vi "bgd squarewave.vi"(9 "YScale.Maximum":dbl, 10 "ZScale.Maximum":dbl, 11 "Cond. Intens. 2":dbl[][](graph)) -> (3 "square wave":dbl[][](array[numeric]))   [LabVIEW 2016]
uses:
  <vilib>/Analysis/NI_AALBase.lvlib
panel:
  in  "place on color scale":dbl(slide)=3.25 scale=0.0..10.0
  in  "color difference":dbl(slide)=8.0 scale=0.0..10.0
  out "Cond. Intens. 3":dbl[][](graph)
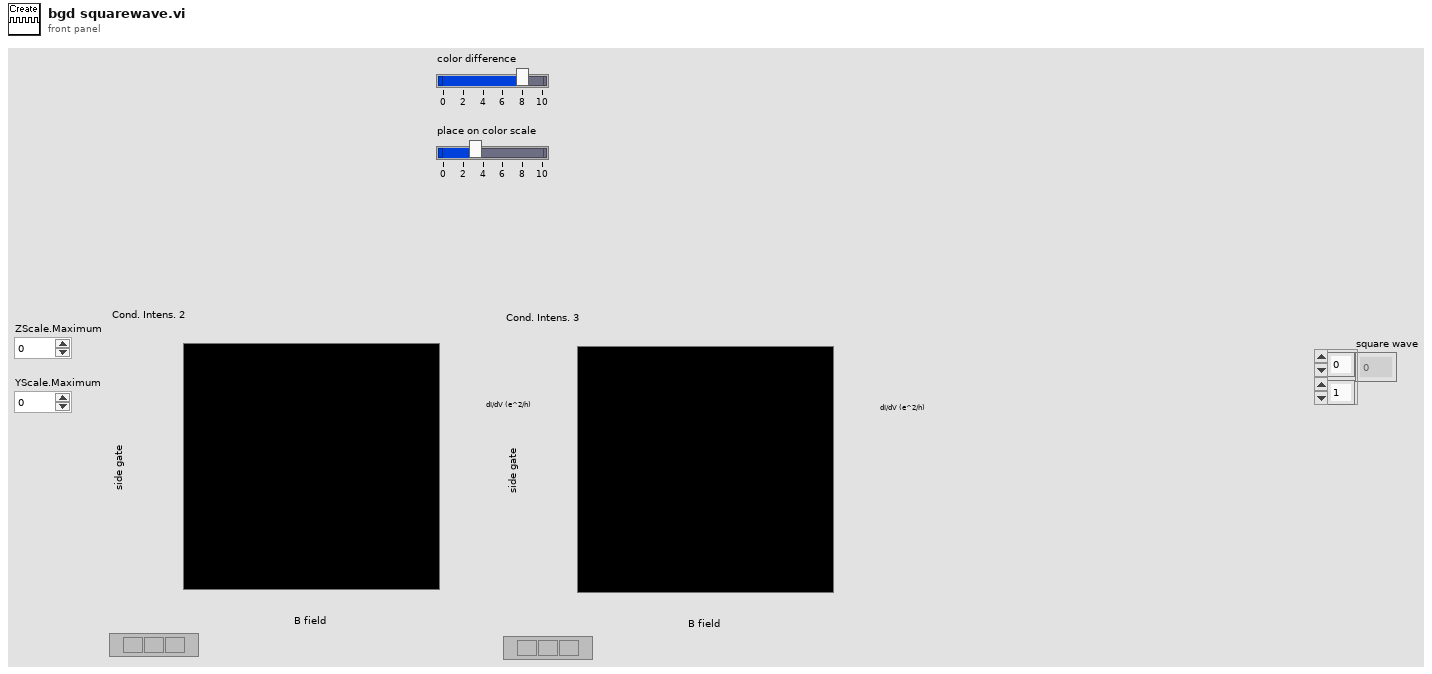
[diagram p1: front panel]
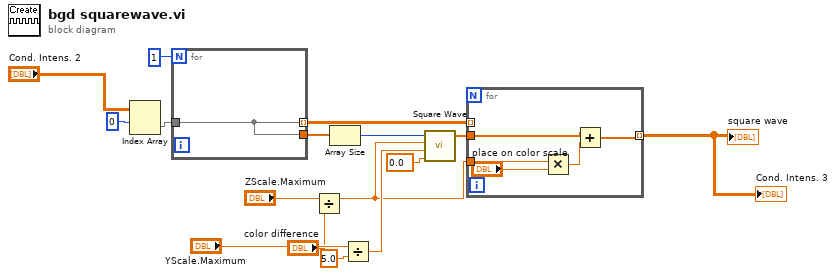
[diagram p0: block diagram]
diagram:
  n1 = Index Array(array="Cond. Intens. 2", index (row)=0 ("index")) -> (element=w8:dbl[])  [unwired: 1 in]
  n2 = for {
    N: 1 -> [_]
    tunnel: w8 -> [w17]
    tunnel: [w17] -> w12
    tunnel: [w17] -> w4 mode=indexing
  }
  n3 = Divide(x="ZScale.Maximum", y="color difference") -> (x/y=w2:dbl)
  n4 = Array Size(array=w12) -> (size(s)=w10:i32)
  n5 = Divide(x="YScale.Maximum", y=5.0) -> (x/y=w14:dbl)
  n6 = call <vilib>:"Square Wave.vi"("samples"=w10, "amplitude"=w2, "frequency"=w14, "phase in"=0.0) -> ("square wave"=w11:dbl[])  [unwired: 2 in, 2 out]
  n7 = for {
    tunnel: w11 -> [w19]
    tunnel: [w18] -> w1 mode=indexing
    tunnel: w4 -> [_] mode=indexing
    tunnel: w2 -> [w20]
    n8 = Multiply(x=w20, y="place on color scale") -> (x*y=w21:dbl)
    n9 = Add(x=w19, y=w21) -> (x+y=w18:dbl[])
  }
  "square wave" <- w1
  "Cond. Intens. 3" <- w1
